vi "readDoubleKey.vi"(0 "Refnum in":T1, 1 "Section":string, 2 "Key Name":string, 3 "error in (no error)":errorcluster) -> (7 "value":dbl, 8 "Warning":string, 10 "error out":errorcluster)   [LabVIEW 2014]
uses:
  <vilib>/Utility/config.llb/Config Data RefNum.ctl
  <vilib>/Utility/config.llb/Read Key (Double).vi
  <vilib>/Utility/config.llb/Write Key (Double).vi
  <vilib>/Utility/config.llb/NI_LVConfig.lvlib
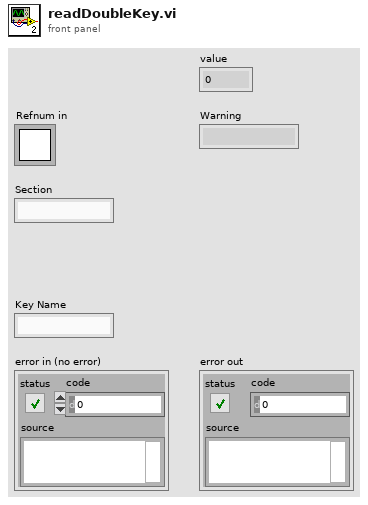
[diagram p1: front panel]
types:
  T1 = typedef "NI_LVConfig.lvlib/Config Data RefNum.ctl" = refnum<k1>
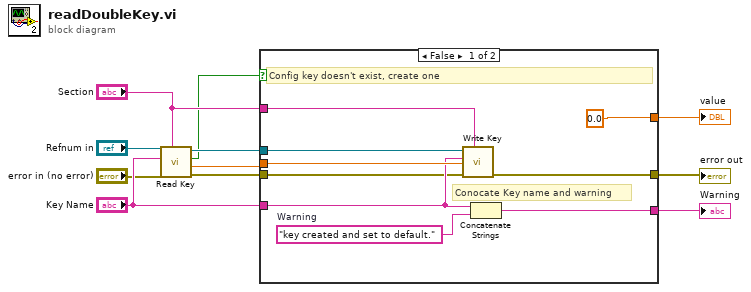
[diagram p0: block diagram]
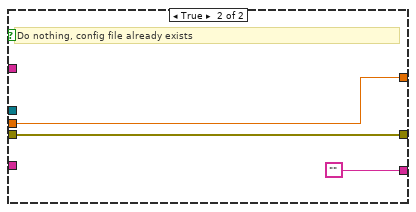
[diagram p2: hidden frame]
diagram:
  n1 = call-poly <vilib>:"Read Key.vi"("section"="Section", "error in (no error)"="error in (no error)", "key"="Key Name", "refnum"="Refnum in") -> ("error out"=w3:errorcluster, "value"=w2:dbl, "found?"=w1:bool, "refnum out"=w6:T1)  [unwired: 4 in]
  n2 = case shown="False" w1 {
    tunnel: w6 -> [w20 _]
    tunnel: "Key Name" -> [w14 _]
    tunnel: w2 -> [w17 w23]
    tunnel: "Section" -> [w19 _]
    tunnel: [w18 w21] -> w5
    tunnel: [0.0 ("value") w23] -> w11
    tunnel: [w13 ""] -> w10
    tunnel: w3 -> [w12 w21]
    frame False {
      w15 = "key created and set to default."  # Warning
      # "Config key doesn't exist, create one"
      # "Conocate Key name and warning"
      n3 = call-poly <vilib>:"Write Key.vi"("section"=w19, "error in (no error)"=w12, "value"=w17, "key"=w14, "refnum"=w20) -> ("error out"=w18:errorcluster)  [unwired: 4 in, 2 out]
      n4 = Concatenate Strings(w14, w15) -> (w13:string)
    }
    frame True {
      # "Do nothing, config file already exists"
    }
  }
  "Warning" <- w10
  "value" <- w11
  "error out" <- w5
